vi "1D experiment_v1199.vi"() -> ()   [LabVIEW 2010]
uses:
  <vilib>/Utility/cursorutil.llb/Set Cursor (Cursor ID).vi
  User32.dll
panel:
  out "1D Experiment":cluster{"Y":dbl[], "Y":dbl[]}[](graph)
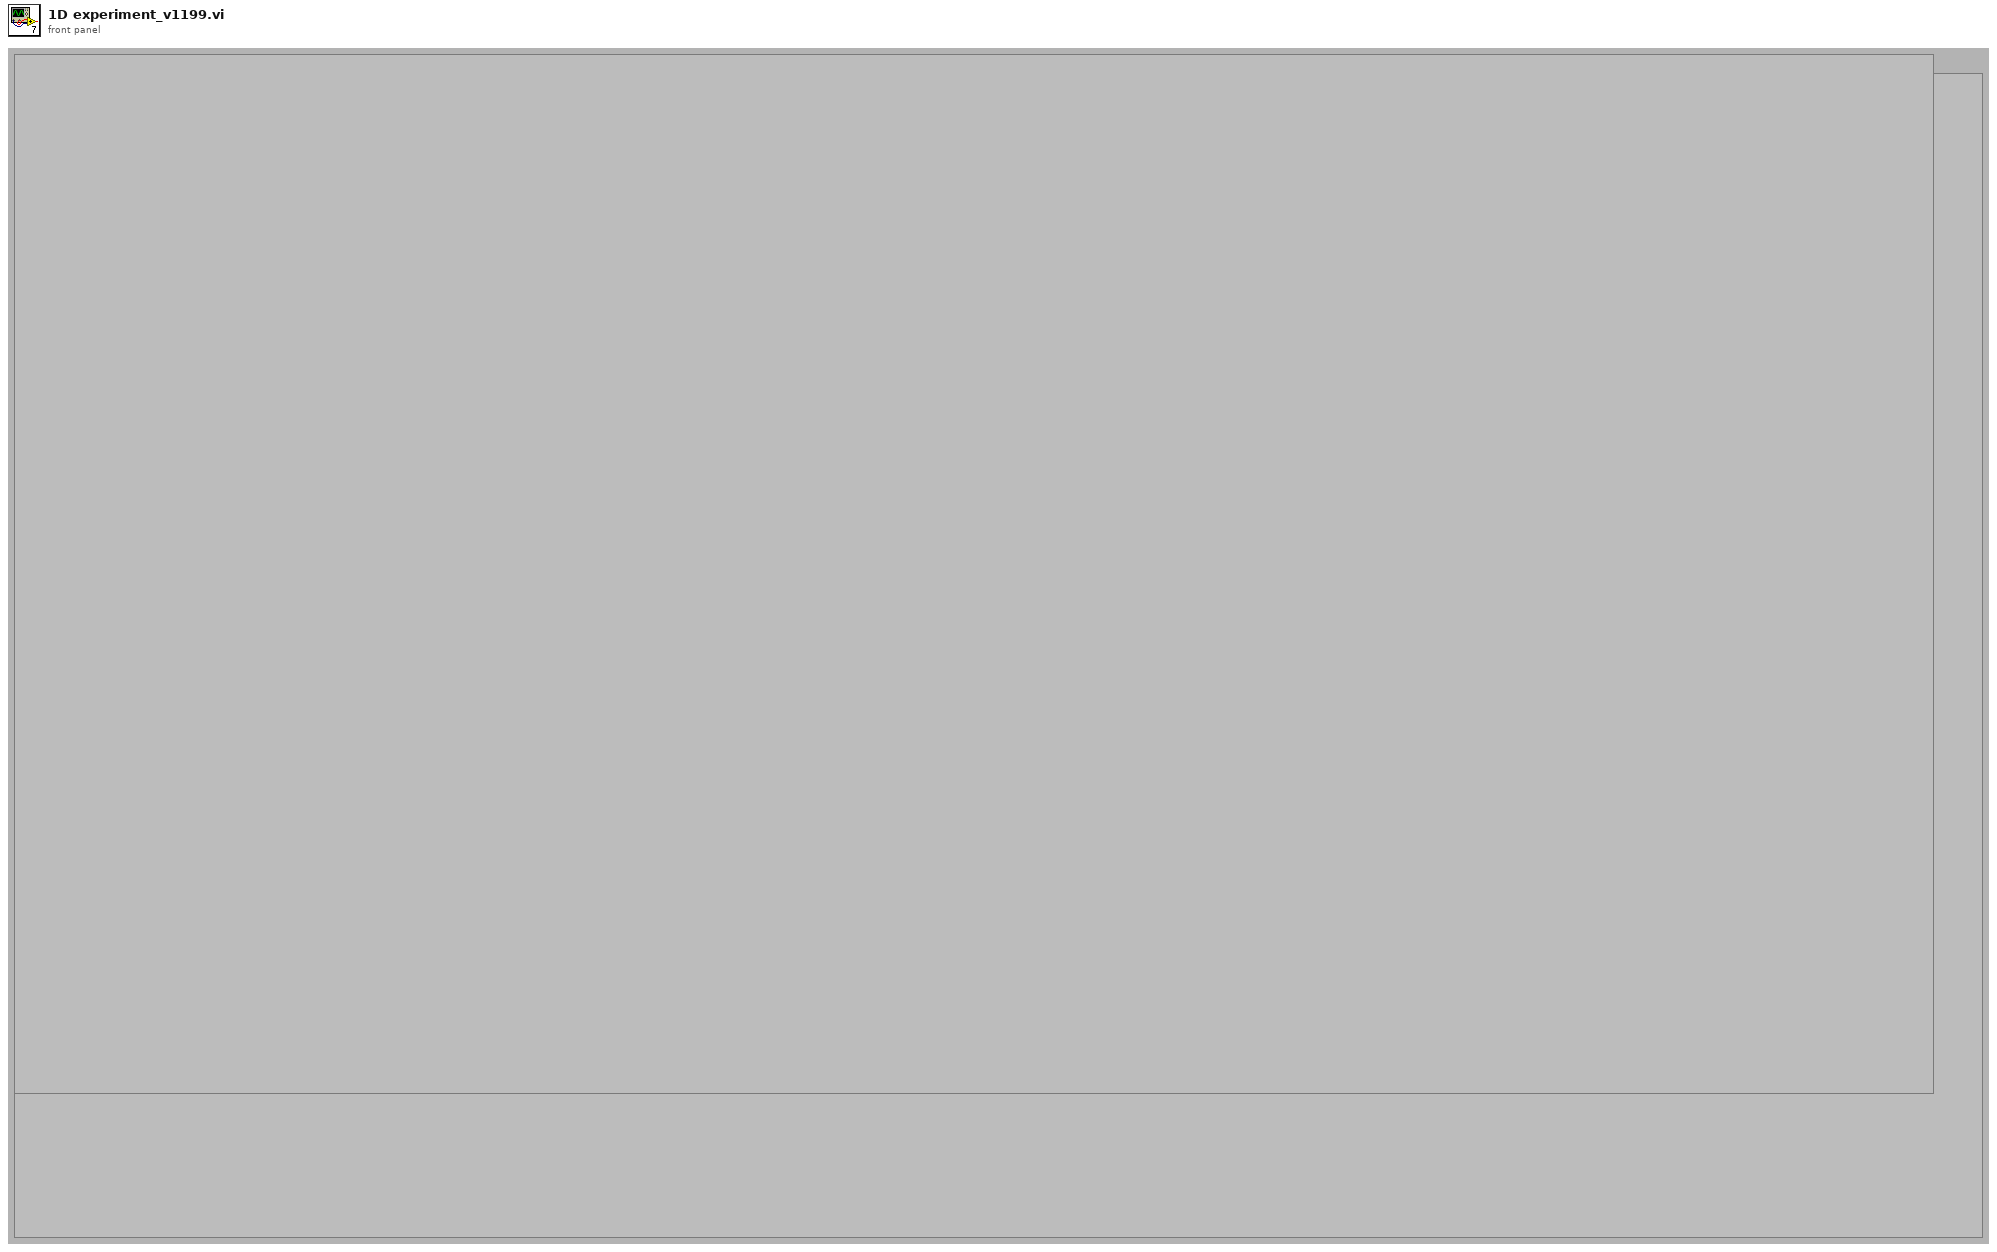
[diagram p1: front panel]
types:
  T1 = cluster{"Radius":dbl, "Center":dbl, "D":dbl, "Valid":bool}
  T2 = typedef "LVAllMonitorsDisplayTypeDef.ctl" = cluster{"Bounds":cluster{"Left":i16, "Top":i16, "Right":i16, "Bottom":i16}, "Depth":i16}[]
  T3 = cluster{"Bounds":cluster{"Left":i16, "Top":i16, "Right":i16, "Bottom":i16}, "Depth":i16}
  T4 = cluster{"Left":i16, "Top":i16, "Right":i16, "Bottom":i16}
  T5 = typedef "Wiimote Buttons.ctl" = cluster{"D-Pad Left":bool, "D-Pad Right":bool, "D-Pad Down":bool, "D-Pad Up":bool, "Plus":bool, "Two":bool, "One":bool, "B":bool, "A":bool, "Minus":bool, "Home":bool}
  T6 = typedef "Wiimote Acceleration.ctl" = cluster{"Acceleration X":dbl, "Acceleration Y":dbl, "Acceleration Z":dbl}
  T7 = typedef "Wiimote IR Sensor.ctl" = cluster{"Point 1":T8, "Point 2":T8, "Point 3":T8, "Point 4":T8}
  T8 = typedef "Wiimote Point.ctl" = cluster{"X":u16, "Y":u16}
  T9 = typedef "Nunchuk Buttons.ctl" = cluster{"C":bool, "Z":bool}
  T10 = cluster{"Wiimote Buttons":T5, "Wiimote Acceleration Raw":T6, "Wiimote IR Sensor":T7, "Nunchuk Analog Stick":T8, "Nunchuk Acceleration Raw":T6, "Nunchuk Buttons":T9}
  T11 = typedef "LVPoint32TypeDef.ctl" = cluster{"Horizontal":i32, "Vertical":i32}
  T12 = cluster{"Cursor.Cursor Position:Cursor X":dbl, "Cursor.Cursor Position:Cursor X":dbl}
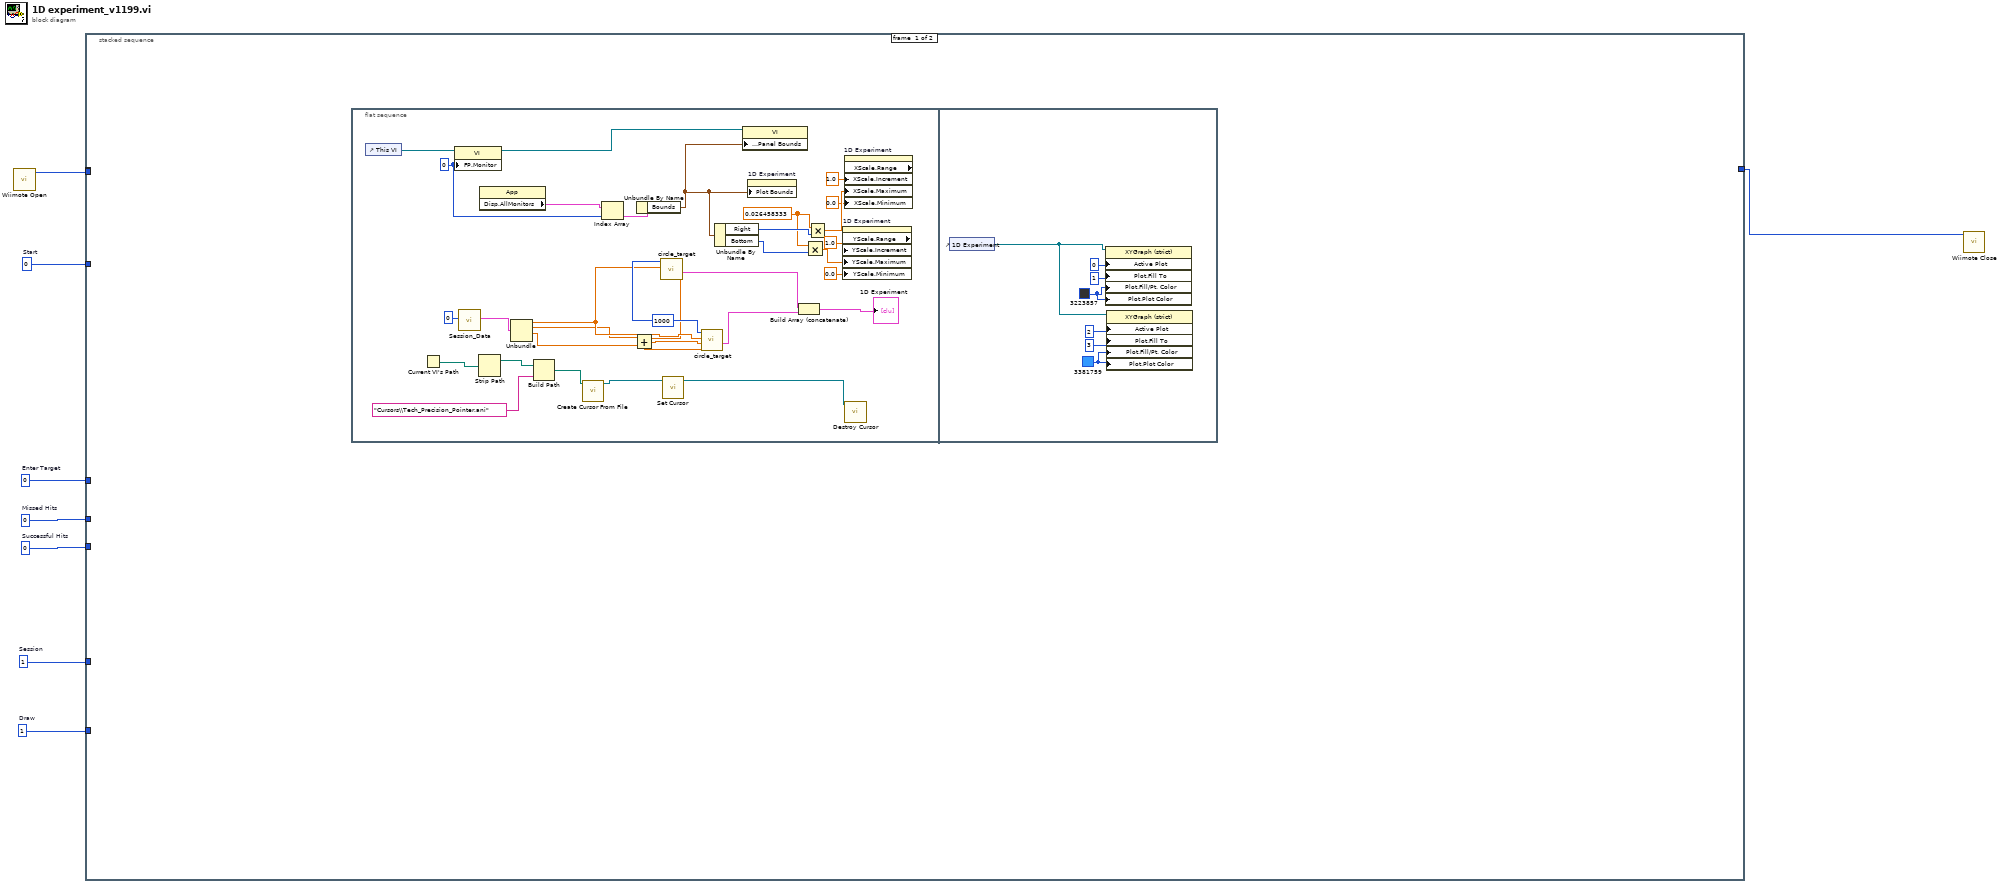
[diagram p0: block diagram]
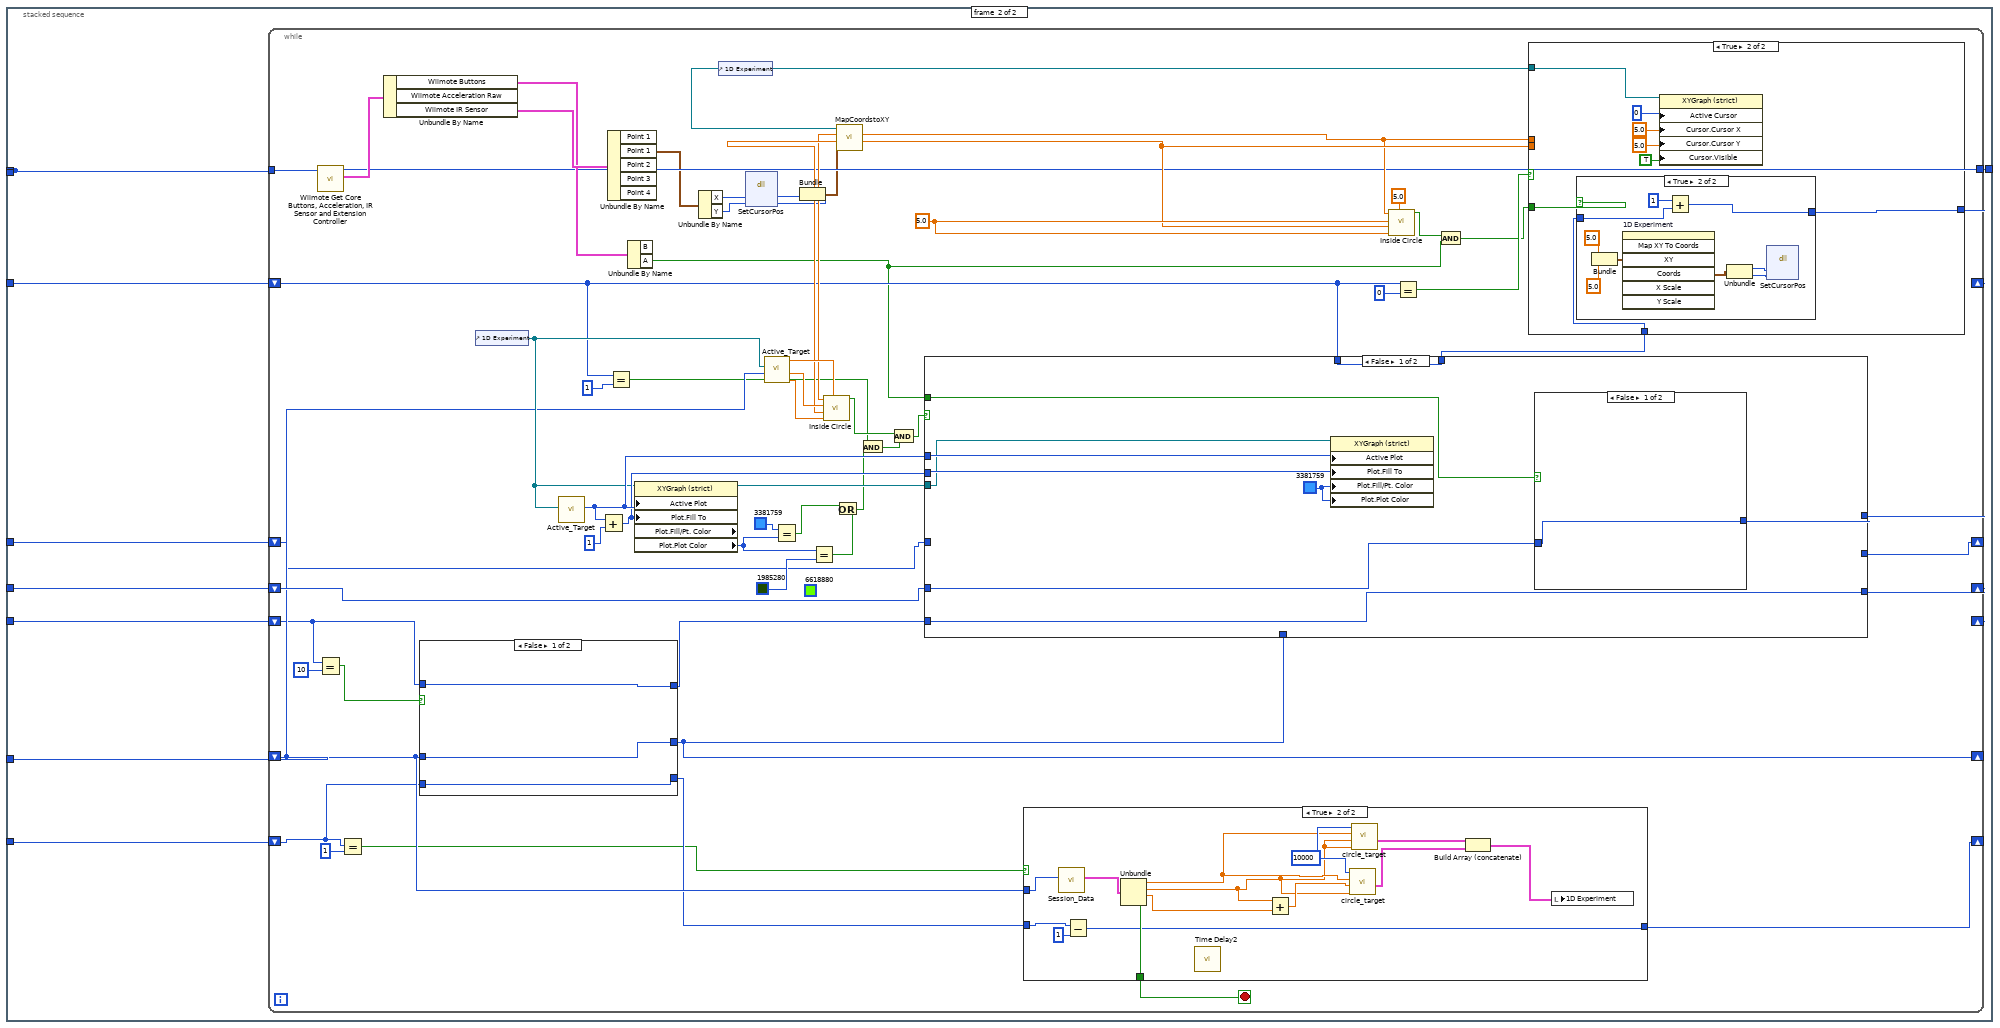
[diagram p2: hidden frame]
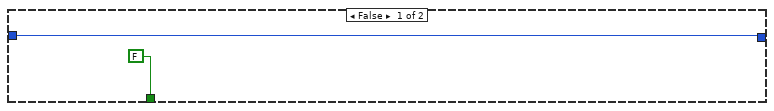
[diagram p3: hidden frame]
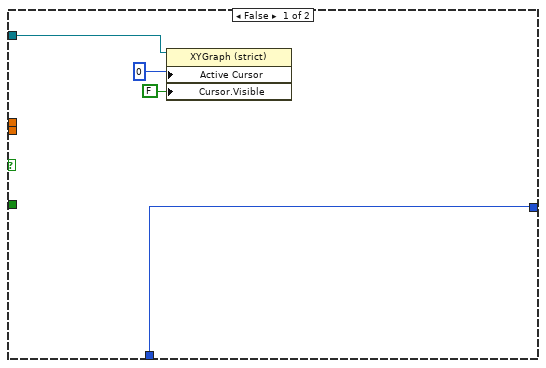
[diagram p4: hidden frame]
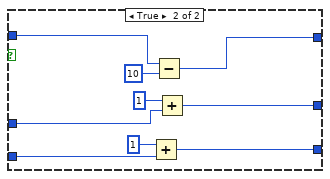
[diagram p6: hidden frame]
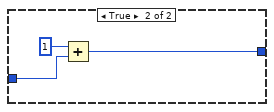
[diagram p7: hidden frame]
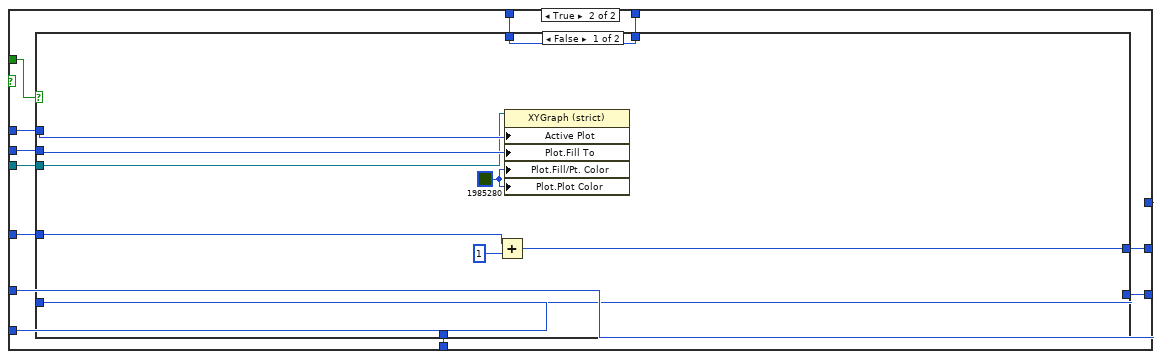
[diagram p8: hidden frame]
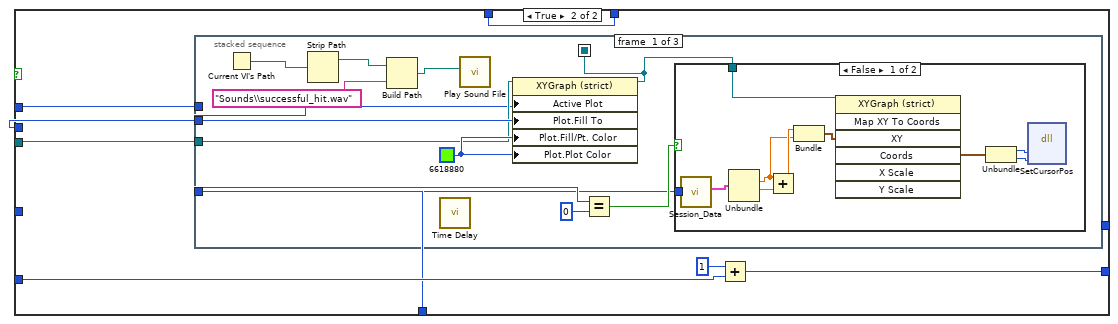
[diagram p9: hidden frame]
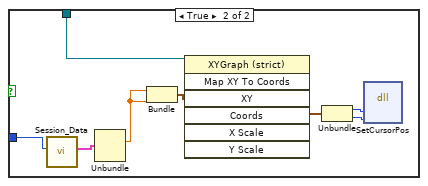
[diagram p10: hidden frame]
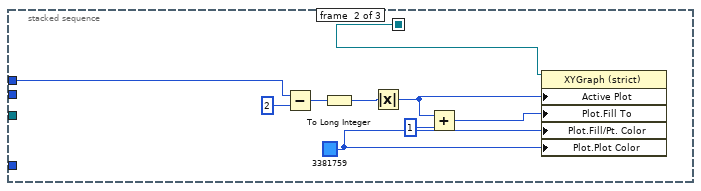
[diagram p11: hidden frame]
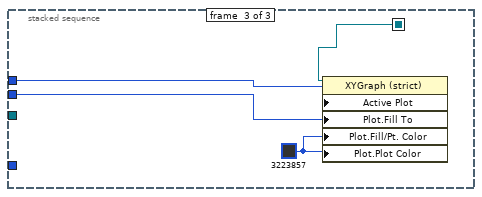
[diagram p12: hidden frame]
diagram:
  w3 = 0  # Enter Target
  w4 = 1  # Draw
  w5 = 0  # Start
  w6 = 1  # Session
  w7 = 0  # Missed Hits
  w8 = 0  # Successful Hits
  n1 = call "Wiimote Open.vi"() -> ("hWiimoteHandle"=w2:u32)  [unwired: 10 in, 1 out]
  n2 = stacked-sequence {
    tunnel: [_ w48] -> _
    tunnel: w8 -> [_ w54]
    tunnel: w7 -> [_ w53]
    tunnel: w6 -> [_ w52]
    tunnel: w5 -> [_ w51]
    tunnel: w4 -> [_ w50]
    tunnel: w3 -> [_ w49]
    tunnel: w2 -> [_ w48]
    tunnel: [_ w47] -> w1
    frame #0 {
      n3 = flat-sequence {
        frame #0 {
          w16 = 0.026458333 ("y")
          w27 = u16 0 ("Front Panel Window:Monitor")
          w39 = 1000
          n4 = control-ref of="This VI"() -> (w29:refnum<vi>)
          n5 = Current VI's Path() -> (path=w24:path)
          n6 = property class="VI"(reference=w29, "FP.Monitor"=w27) -> (reference out=w25:refnum<vi>)  [unwired: 1 in, 1 out]
          n7 = call "Session_Data.vi"("Session"=0) -> ("output cluster"=w37:T1)  [unwired: 10 in]
          n8 = Strip Path(path=w24) -> (stripped path=w23:path)  [unwired: 1 out]
          n9 = property class="App"() -> ("Disp.AllMonitors"=w26:T2)  [unwired: 2 in, 2 out]
          n10 = Unbundle(w37) -> ("Radius"=w36:dbl, "Center"=w34:dbl, "D"=w35:dbl)  [unwired: 1 out]
          n11 = Build Path(base path=w23, name or relative path="Cursors\\Tech_Precision_Pointer.ani") -> (appended path=w21:path)
          n12 = call <vilib>:"Create Cursor From File.vi"("cursor file"=w21) -> ("cursor ID"=w20:refnum<k1>)  [unwired: 9 in, 1 out]
          n13 = Index Array(array=w26, index=w27) -> (element=w28:T3)
          n14 = Add(x=w34, y=w35) -> (x+y=w38:dbl)
          n15 = Unbundle By Name(w28) -> ("Bounds"=w18:T4)
          n16 = call "circle_target.vi"("y0"=w34, "x0"=w34, "Radius"=w36, "Pixels"=w39) -> ("Target plots"=w32:cluster{dbl[], dbl[]}[])  [unwired: 7 in]
          n17 = call-poly <vilib>:"Set Cursor.vi"("cursor ID"=w20) -> ("previous cursor ID"=w19:refnum<k1>)  [unwired: 9 in, 1 out]
          n18 = call "circle_target.vi"("y0"=w34, "x0"=w38, "Radius"=w36, "Pixels"=w39) -> ("Target plots"=w33:cluster{dbl[], dbl[]}[])  [unwired: 7 in]
          n19 = Unbundle By Name(w18) -> ("Right"=w17:i16, "Bottom"=w15:i16)
          n20 = property class="VI"(reference=w25, "Front Panel Window:Panel Bounds"=w18) -> ()  [unwired: 1 in, 2 out]
          n21 = property on="1D Experiment" class="XYGraph (strict)"("Plot Bounds"=w18) -> ()  [unwired: 2 in, 2 out]
          n22 = Build Array (concatenate)(w32, w33) -> (→"1D Experiment":cluster{dbl[], dbl[]}[])
          n23 = Multiply(x=w16, y=w15) -> (x*y=w10:dbl)
          n24 = Multiply(x=w16, y=w17) -> (x*y=w13:dbl)
          n25 = property on="1D Experiment" class="XYGraph (strict)" props=["YScale", "Range", "YScale", "Increment", "YScale", "Maximum", "YScale", "Minimum"]("YScale.Increment"=1.0 ("Y Scale.Range:Increment"), "YScale.Maximum"=w10, "YScale.Minimum"=0.0 ("Y Scale.Range:Minimum")) -> ()  [unwired: 2 in, 3 out]
          n26 = property on="1D Experiment" class="XYGraph (strict)" props=["XScale", "Range", "XScale", "Increment", "XScale", "Maximum", "XScale", "Minimum"]("XScale.Increment"=1.0 ("X Scale.Range:Increment"), "XScale.Maximum"=w13, "XScale.Minimum"=0.0 ("X Scale.Range:Minimum")) -> ()  [unwired: 2 in, 3 out]
          n27 = call <vilib>:"Destroy Cursor.vi"("cursor ID"=w19) -> ()  [unwired: 9 in, 1 out]
        }
        frame #1 {
          w45 = u32 3381759
          w42 = u32 3223857
          n28 = control-ref of="1D Experiment"() -> (w46:refnum<vi>)
          n29 = property on="Property Node" class="XYGraph (strict)"(reference=w46, "Active Plot"=u32 0, "Plot.Fill To"=i16 1, "Plot.Fill/Pt. Color"=w42, "Plot.Plot Color"=w42) -> ()  [unwired: 1 in, 2 out]
          n30 = property on="Property Node" class="XYGraph (strict)"(reference=w46, "Active Plot"=u32 2, "Plot.Fill To"=i16 3, "Plot.Fill/Pt. Color"=w45, "Plot.Plot Color"=w45) -> ()  [unwired: 1 in, 2 out]
        }
      }
    }
    frame #1 {
      n31 = while {
        tunnel: w48 -> [w66]
        shift-right: [w104] -> _
        shift-left: w54 -> [w84]
        shift-right: [w102] -> _
        shift-left: w53 -> [w103]
        shift-right: [w76] -> _
        shift-left: w52 -> [w85]
        shift-right: [w90] -> _
        shift-left: w51 -> [w73]
        shift-right: [w81] -> _
        shift-left: w50 -> [w82]
        shift-right: [w77] -> _
        shift-left: w49 -> [w78]
        tunnel: [w62] -> w47
        stop <- w86 stop-if-true
        (unwired) u32 6618880
        w94 = 5.0 ("x0")
        n32 = call "Wiimote Get Core Buttons, Acceleration, IR Sensor and Extension Controller.vi"("hWiimoteHandle in"=w66) -> ("Data out"=w65:T10, "hWiimoteHandle out"=w62:u32)  [unwired: 8 in, 1 out]
        n33 = Equal?(x=w84, y=10) -> (x = y?=w100:bool)
        n34 = Equal?(x=w82, y=1) -> (x = y?=w79:bool)
        n35 = Unbundle By Name(w65) -> ("Wiimote Buttons"=w63:T5, "Wiimote IR Sensor"=w64:T7)  [unwired: 1 out]
        n36 = case shown="False" w100 {
          tunnel: w84 -> [w155 w164]
          tunnel: [w155 w162] -> w99
          tunnel: w85 -> [w154 w161]
          tunnel: [w154 w159] -> w76
          tunnel: w82 -> [w153 w158]
          tunnel: [w153 w156] -> w80
          frame False {
          }
          frame True {
            n37 = Add(x=1, y=w158) -> (x+y=w156:i32)
            n38 = Subtract(x=w164, y=10) -> (x-y=w162:i32)
            n39 = Add(x=1, y=w161) -> (x+y=w159:i32)
          }
        }
        n40 = control-ref of="1D Experiment"() -> (w97:refnum<vi>)
        n41 = call "Active_Target.vi"("XYGraph Refnum"=w97) -> ("Active Plot"=w108:u32)  [unwired: 7 in, 3 out]
        n42 = Add(x=w108, y=u32 1) -> (x+y=w107:u32)
        n43 = Unbundle By Name(w64) -> ("Point 1"=w61:T8)  [unwired: 4 out]
        n44 = Equal?(x=w73, y=1) -> (x = y?=w69:bool)
        n45 = Unbundle By Name(w63) -> ("A"=w55:bool)  [unwired: 1 out]
        n46 = property on="Property Node" class="XYGraph (strict)" props=["Active Plot", "Plot", "Fill To", "Plot", "Fill/Pt. Color", "Plot", "Plot Color"](reference=w97, "Active Plot"=w108, "Plot.Fill To"=w107) -> (reference out=w87:refnum<vi>, "Plot.Plot Color"=w89:u32)  [unwired: 1 in, 2 out]
        n47 = Unbundle By Name(w61) -> ("X"=w60:u16, "Y"=w59:u16)
        n48 = control-ref of="1D Experiment"() -> (w67:refnum<vi>)
        n49 = dll-call lib="User32.dll" fn="SetCursorPos"(w60, w59) -> (w58:i32, w57:i32)  [unwired: 4 in, 2 out]
        n50 = call "Active_Target.vi"("Session"=w85, "XYGraph Refnum"=w97) -> ("y0"=w105:dbl, "x0"=w106:dbl, "Radius"=w98:dbl)  [unwired: 6 in, 1 out]
        n51 = Equal?(x=u32 3381759, y=w89) -> (x = y?=w111:bool)
        n52 = Bundle(w58, w57) -> (w56:cluster{i32, i32})  [unwired: 1 in]
        n53 = Equal?(x=w89, y=u32 1985280) -> (x = y?=w110:bool)
        n54 = Or(x=w111, y=w110) -> (x .or. y?=w71:bool)
        n55 = call "MapCoordstoXY.vi"("Coordinates"=w56, "XYGraph Refnum"=w67) -> ("Y(graph)"=w75:dbl, "X (graph)"=w74:dbl)  [unwired: 7 in]
        n56 = call "Inside Circle.vi"("Radius"=w98, "y0"=w105, "y"=w75, "x0"=w106, "x"=w74) -> ("Inside Circle"=w70:bool)  [unwired: 6 in]
        n57 = And(x=w69, y=w71) -> (x .and. y?=w68:bool)
        n58 = And(x=w70, y=w68) -> (x .and. y?=w113:bool)
        n59 = case shown="False" w113 {
          tunnel: w55 -> [w171 w189]
          tunnel: w108 -> [w168 w185]
          tunnel: w107 -> [w167 w184]
          tunnel: w99 -> [w172 w188]
          tunnel: [w172 w187] -> w104
          tunnel: w103 -> [w170 w186]
          tunnel: [w169 w186] -> w102
          tunnel: w73 -> [w166 w183]
          tunnel: [w166 w182] -> w88
          tunnel: w87 -> [w165 w181]
          tunnel: w78 -> [_ w180]
          tunnel: [_ w179] -> w77
          tunnel: w76 -> [_ w178]
          frame False {
            w173 = u32 3381759
            n60 = property on="Property Node" class="XYGraph (strict)"(reference=w165, "Active Plot"=w168, "Plot.Fill To"=w167, "Plot.Fill/Pt. Color"=w173, "Plot.Plot Color"=w173) -> ()  [unwired: 1 in, 2 out]
            n61 = case shown="False" w171 {
              tunnel: w170 -> [w174 w177]
              tunnel: [w174 w175] -> w169
              frame False {
              }
              frame True {
                n62 = Add(x=1, y=w177) -> (x+y=w175:i32)
              }
            }
          }
          frame True {
            n63 = case shown="False" w189 {
              tunnel: w188 -> [w197 w206]
              tunnel: [w197 w200] -> w187
              tunnel: w185 -> [w196 w204]
              tunnel: w184 -> [w195 w203]
              tunnel: w183 -> [w194 w202]
              tunnel: [w194 w202] -> w182
              tunnel: w181 -> [w193 w201]
              tunnel: w180 -> [w192 _]
              tunnel: [w190 _] -> w179
              tunnel: w178 -> [_ w199]
              frame False {
                w198 = u32 1985280
                n64 = Add(x=w192, y=1) -> (x+y=w190:i32)
                n65 = property on="Property Node" class="XYGraph (strict)"(reference=w193, "Active Plot"=w196, "Plot.Fill To"=w195, "Plot.Fill/Pt. Color"=w198, "Plot.Plot Color"=w198) -> ()  [unwired: 1 in, 2 out]
              }
              frame True {
                n66 = stacked-sequence {
                  seq-local: [w215 _ _] -> [_ w237 w246]
                  tunnel: w204 -> [w214 w238 w248]
                  tunnel: w203 -> [w217 _ w247]
                  tunnel: w201 -> [w216 _ _]
                  tunnel: w199 -> [w211 _ _]
                  frame #0 {
                    w218 = u32 6618880
                    n67 = Current VI's Path() -> (path=w208:path)
                    n68 = Strip Path(path=w208) -> (stripped path=w207:path)  [unwired: 1 out]
                    n69 = Build Path(base path=w207, name or relative path="Sounds\\successful_hit.wav") -> (appended path=w209:path)
                    n70 = call "Time Delay"() -> ()  [unwired: 11 in, 1 out]
                    n71 = call <vilib>:"Play Sound File.vi"("path"=w209) -> ()  [unwired: 9 in, 2 out]
                    n72 = property on="Property Node" class="XYGraph (strict)"(reference=w216, "Active Plot"=w214, "Plot.Fill To"=w217, "Plot.Fill/Pt. Color"=w218, "Plot.Plot Color"=w218) -> (reference out=w215:refnum<vi>)  [unwired: 1 in, 1 out]
                    n73 = Equal?(x=w214, y=u32 0) -> (x = y?=w212:bool)
                    n74 = case shown="False" w212 {
                      tunnel: w215 -> [w224 w229]
                      tunnel: w211 -> [w221 w233]
                      frame False {
                        n75 = call "Session_Data.vi"("Session"=w221) -> ("output cluster"=w225:T1)  [unwired: 10 in]
                        n76 = Unbundle(w225) -> ("Center"=w219:dbl, "D"=w223:dbl)  [unwired: 2 out]
                        n77 = Add(x=w219, y=w223) -> (x+y=w220:dbl)
                        n78 = Bundle(w220, "Center"=w219) -> (w222:cluster{dbl, "Center":dbl})  [unwired: 1 in]
                        n79 = invoke on="Invoke Node" class="XYGraph (strict)" method="Map XY To Coords"(reference=w224, "XY"=w222) -> ("Coords"=w228:T11)  [unwired: 5 in, 6 out]
                        n80 = Unbundle(w228) -> ("Horizontal"=w227:i32, "Vertical"=w226:i32)
                        n81 = dll-call lib="User32.dll" fn="SetCursorPos"(w227, w226) -> ()  [unwired: 6 in, 2 out]
                      }
                      frame True {
                        n82 = call "Session_Data.vi"("Session"=w233) -> ("output cluster"=w232:T1)  [unwired: 10 in]
                        n83 = Unbundle(w232) -> ("Center"=w231:dbl)  [unwired: 3 out]
                        n84 = Bundle("Center"=w231, "Center"=w231) -> (w230:cluster{"Center":dbl, "Center":dbl})  [unwired: 1 in]
                        n85 = invoke on="Invoke Node" class="XYGraph (strict)" method="Map XY To Coords"(reference=w229, "XY"=w230) -> ("Coords"=w236:T11)  [unwired: 5 in, 6 out]
                        n86 = Unbundle(w236) -> ("Horizontal"=w235:i32, "Vertical"=w234:i32)
                        n87 = dll-call lib="User32.dll" fn="SetCursorPos"(w235, w234) -> ()  [unwired: 6 in, 2 out]
                      }
                    }
                  }
                  frame #1 {
                    w245 = u32 3381759
                    n88 = Subtract(x=w238, y=u32 2) -> (x-y=w242:u32)
                    n89 = To Long Integer(number=w242) -> (32bit integer=w241:i32)
                    n90 = Absolute Value(x=w241) -> (abs(x)=w239:i32)
                    n91 = Add(x=w239, y=u32 1) -> (x+y=w243:u32)
                    n92 = property on="Property Node" class="XYGraph (strict)"(reference=w237, "Active Plot"=w239, "Plot.Fill To"=w243, "Plot.Fill/Pt. Color"=w245, "Plot.Plot Color"=w245) -> ()  [unwired: 1 in, 2 out]
                  }
                  frame #2 {
                    w249 = u32 3223857
                    n93 = property on="Property Node" class="XYGraph (strict)"(reference=w246, "Active Plot"=w248, "Plot.Fill To"=w247, "Plot.Fill/Pt. Color"=w249, "Plot.Plot Color"=w249) -> ()  [unwired: 1 in, 2 out]
                  }
                }
                n94 = Add(x=1, y=w206) -> (x+y=w200:i32)
              }
            }
          }
        }
        n95 = case shown="True" w79 {
          tunnel: [FALSE ("Valid") w122] -> w86
          tunnel: w85 -> [_ w121]
          tunnel: [w115 w119] -> w81
          tunnel: w80 -> [w115 w118]
          frame False {
          }
          frame True {
            w130 = 10000
            n96 = call "Session_Data.vi"("Session"=w121) -> ("output cluster"=w128:T1)  [unwired: 10 in]
            n97 = Subtract(x=w118, y=1) -> (x-y=w119:i32)
            n98 = Unbundle(w128) -> ("Radius"=w127:dbl, "Center"=w125:dbl, "D"=w126:dbl, "Valid"=w122:bool)
            n99 = call "Time Delay2"() -> ()  [unwired: 11 in, 1 out]
            n100 = Add(x=w125, y=w126) -> (x+y=w129:dbl)
            n101 = call "circle_target.vi"("y0"=w125, "x0"=w129, "Radius"=w127, "Pixels"=w130) -> ("Target plots"=w123:cluster{dbl[], dbl[]}[])  [unwired: 7 in]
            n102 = call "circle_target.vi"("y0"=w125, "x0"=w125, "Radius"=w127, "Pixels"=w130) -> ("Target plots"=w124:cluster{dbl[], dbl[]}[])  [unwired: 7 in]
            n103 = Build Array (concatenate)(w124, w123) -> (w117:cluster{dbl[], dbl[]}[])
            n104 = local write "1D Experiment"(w117) -> ()
          }
        }
        n105 = call "Inside Circle.vi"("Radius"=5.0, "y0"=w94, "y"=w75, "x0"=w94, "x"=w74) -> ("Inside Circle"=w92:bool)  [unwired: 6 in]
        n106 = Equal?(x=w73, y=0) -> (x = y?=w95:bool)
        n107 = And(x=w92, y=w55) -> (x .and. y?=w91:bool)
        n108 = case shown="True" w95 {
          tunnel: w67 -> [w131 w136]
          tunnel: w74 -> [_ _]
          tunnel: w75 -> [_ _]
          tunnel: w91 -> [_ w139]
          tunnel: w88 -> [w134 w138]
          tunnel: [w134 w137] -> w90
          frame False {
            n109 = property on="Property Node" class="XYGraph (strict)"(reference=w131, "Active Cursor"=u32 0, "Cursor.Visible"=FALSE) -> ()  [unwired: 1 in, 2 out]
          }
          frame True {
            n110 = case shown="True" w139 {
              tunnel: w138 -> [w143 w152]
              tunnel: [w143 w150] -> w137
              frame False {
              }
              frame True {
                n111 = Bundle("Cursor.Cursor Position:Cursor X"=5.0, "Cursor.Cursor Position:Cursor X"=5.0) -> (w147:T12)  [unwired: 1 in]
                n112 = invoke on="1D Experiment" class="XYGraph (strict)" method="Map XY To Coords"("XY"=w147) -> ("Coords"=w146:T11)  [unwired: 6 in, 6 out]
                n113 = Add(x=1, y=w152) -> (x+y=w150:i32)
                n114 = Unbundle(w146) -> ("Horizontal"=w145:i32, "Vertical"=w144:i32)
                n115 = dll-call lib="User32.dll" fn="SetCursorPos"(w145, w144) -> ()  [unwired: 6 in, 2 out]
              }
            }
            n116 = property on="Property Node" class="XYGraph (strict)"(reference=w136, "Active Cursor"=u32 0, "Cursor.Cursor X"=5.0 ("Cursor.Cursor Position:Cursor X"), "Cursor.Cursor Y"=5.0 ("Cursor.Cursor Position:Cursor Y"), "Cursor.Visible"=TRUE) -> ()  [unwired: 1 in, 2 out]
          }
        }
      }
    }
  }
  n117 = call "Wiimote Close.vi"("hWiimoteHandle in"=w1) -> ()  [unwired: 10 in, 1 out]
